vi "SetBasePath.vi"(8 "error in (no error)":errorcluster, 10 "base_path":path=path "D:/Sgraph_database", 11 "DBAL-BIN in":refnum<class "DBAL-BIN.lvclass">) -> (0 "error out":errorcluster, 3 "DBAL-BIN out":refnum<class "DBAL-BIN.lvclass">)   [LabVIEW 2020, in "Sgraph_lib_V1.lvlib" / "DBAL-BIN.lvclass"]
doc: "Write Database path"
uses:
  DBAL-BIN.lvclass
  DBAL-BIN.lvclass/DBAL-BIN.ctl
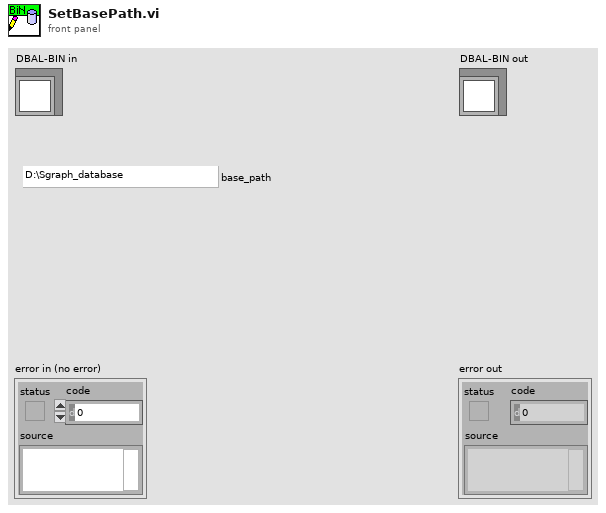
[diagram p1: front panel]
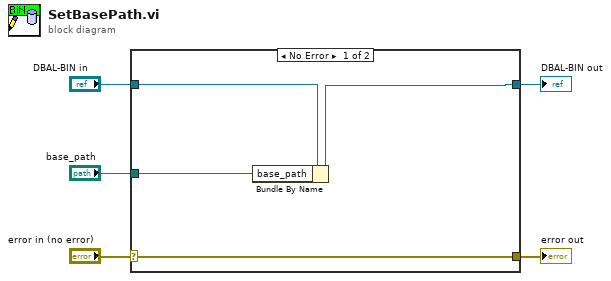
[diagram p0: block diagram]
diagram:
  n1 = case shown="No Error" "error in (no error)" {
    selector: "error in (no error)" -> [w9 w10]
    tunnel: [w9 w10] -> w4
    tunnel: [w7 w11] -> w2
    tunnel: "DBAL-BIN in" -> [w8 w11]
    tunnel: "base_path" -> [w6 _]
    frame No Error {
      n2 = Bundle By Name(cluster=w8, "base_path"=w6) -> (w7:refnum<class "DBAL-BIN.lvclass">)
    }
    frame Error {
    }
  }
  "error out" <- w4
  "DBAL-BIN out" <- w2
